vi "ZoneVacCtrldPickDrop_2StepVac.vi"(4 "Position":enum16{"1", "2"}(ring), 5 "VacuumState2":u8, 6 "Zone":enum16{"ZoneA", "ZoneB", "ZoneC", "ZoneD"}(ring), 7 "VacuumState1":u8, 8 "error in (no error)":errorcluster, 9 "controller in":refnum<k24>, 10 "Zspeed":dbl=50.0 format="%#_13g", 11 "Z":dbl=65.0) -> (0 "error out":errorcluster, 3 "controller out":refnum<k24>)   [LabVIEW 2019]
uses:
  C:/Users/TTUHEP/Documents/LabVIEW/Other Models/2010/Bin/Aerotech.A3200.dll
  Other Models/2010/Bin/Aerotech.A3200.dll
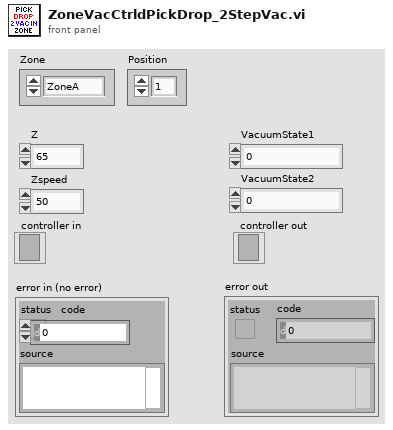
[diagram p1: front panel]
types:
  T1 = enum16{"BinarySwitch", "DecimalSwitch", "Conversion"}
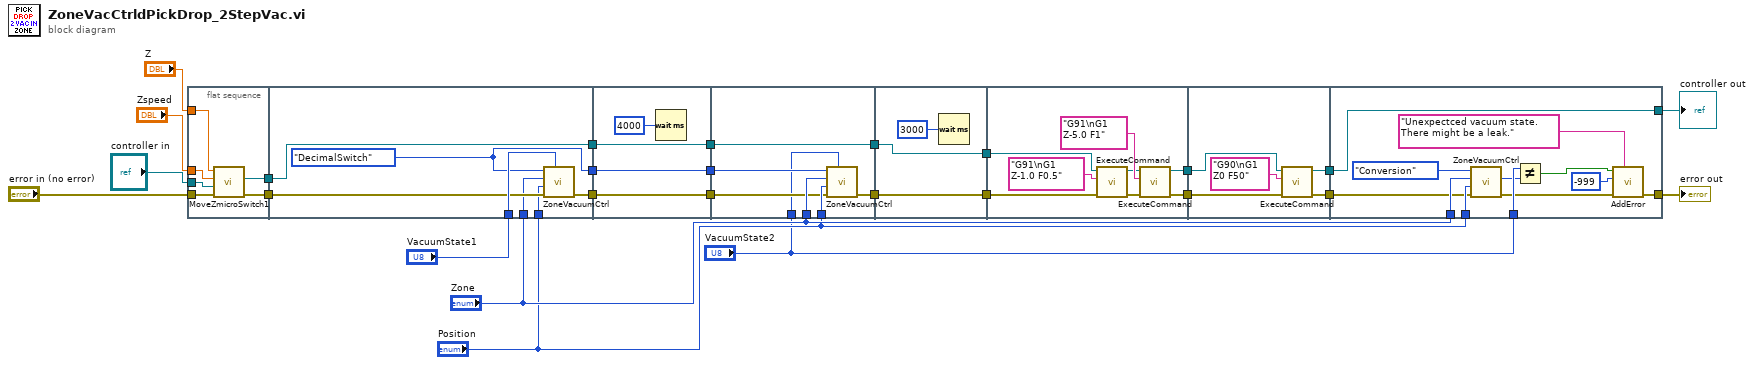
[diagram p0: block diagram]
diagram:
  n1 = flat-sequence {
    tunnel: [w29] -> w13
    tunnel: [w30] -> w12
    tunnel: "controller in" -> [w32]
    tunnel: "error in (no error)" -> [w31]
    tunnel: "Z" -> [w28]
    tunnel: "Zspeed" -> [w27]
    tunnel: w13 -> [w37]
    tunnel: [w34] -> w22
    tunnel: [w39] -> w21
    tunnel: w12 -> [w39]
    tunnel: "VacuumState1" -> [w38]
    tunnel: "Position" -> [w36]
    tunnel: "Zone" -> [w35]
    tunnel: [w33] -> w9
    tunnel: w22 -> [w43]
    tunnel: [w43] -> w11
    tunnel: w21 -> [w42]
    tunnel: [w42] -> w10
    tunnel: w9 -> [w40]
    tunnel: [w40] -> w8
    tunnel: w11 -> [w46]
    tunnel: [w45] -> w5
    tunnel: w10 -> [w50]
    tunnel: [w50] -> w3
    tunnel: w8 -> [w49]
    tunnel: "Zone" -> [w48]
    tunnel: "Position" -> [w47]
    tunnel: "VacuumState2" -> [w44]
    tunnel: w5 -> [w53]
    tunnel: [w53] -> w4
    tunnel: w3 -> [w52]
    tunnel: [w52] -> w2
    tunnel: w4 -> [w59]
    tunnel: [w54] -> w17
    tunnel: w2 -> [w60]
    tunnel: [w55] -> w16
    tunnel: w17 -> [w66]
    tunnel: w16 -> [w64]
    tunnel: [w63] -> w20
    tunnel: [w62] -> w14
    tunnel: w20 -> [w75]
    tunnel: [w76] -> w19
    tunnel: [w75] -> w18
    tunnel: "VacuumState2" -> [w74]
    tunnel: w14 -> [w70]
    tunnel: "Position" -> [w73]
    tunnel: "Zone" -> [w72]
    frame #0 {
      n2 = call "MoveZmicroSwitch1.vi"("Z"=w28, "Zspeed"=w27, "controller in"=w32, "error in (no error)"=w31) -> ("controller out"=w30:refnum<k24>, "error out"=w29:errorcluster)  [unwired: 3 in, 2 out]
    }
    frame #1 {
      w33 = T1."DecimalSwitch" ("ControlType")
      n3 = call "ZoneVacuumCtrl.vi"("DecimalIn"=w38, "Error In"=w37, "Position"=w36, "Zone"=w35, "ControlType"=w33) -> ("Error Out"=w34:errorcluster)  [unwired: 2 in, 4 out]
    }
    frame #2 {
      n4 = Wait (ms)(milliseconds to wait=u32 4000) -> ()  [unwired: 1 out]
    }
    frame #3 {
      n5 = call "ZoneVacuumCtrl.vi"("DecimalIn"=w44, "Error In"=w46, "Position"=w47, "Zone"=w48, "ControlType"=w49) -> ("Error Out"=w45:errorcluster)  [unwired: 2 in, 4 out]
    }
    frame #4 {
      n6 = Wait (ms)(milliseconds to wait=u32 3000) -> ()  [unwired: 1 out]
    }
    frame #5 {
      n7 = call "ExecuteCommand.vi"("error in (no error)"=w59, "Command Code"="G91\nG1 Z-1.0 F0.5", "controller in"=w60) -> ("error out"=w56:errorcluster, "controller out"=w57:refnum<k24>)  [unwired: 6 in, 1 out]
      n8 = call "ExecuteCommand.vi"("error in (no error)"=w56, "Command Code"="G91\nG1 Z-5.0 F1", "controller in"=w57) -> ("error out"=w54:errorcluster, "controller out"=w55:refnum<k24>)  [unwired: 6 in, 1 out]
    }
    frame #6 {
      n9 = call "ExecuteCommand.vi"("error in (no error)"=w66, "Command Code"="G90\nG1 Z0 F50", "controller in"=w64) -> ("error out"=w62:errorcluster, "controller out"=w63:refnum<k24>)  [unwired: 6 in, 1 out]
    }
    frame #7 {
      n10 = call "ZoneVacuumCtrl.vi"("Error In"=w70, "Position"=w73, "Zone"=w72, "ControlType"=T1."Conversion") -> ("Error Out"=w71:errorcluster, "DecimalOut"=w68:u32)  [unwired: 3 in, 3 out]
      n11 = Not Equal?(x=w74, y=w68) -> (x != y?=w67:bool)
      n12 = call "AddError.vi"("ErrorMessage"="Unexpectced vacuum state. There might be a leak.", "error in"=w71, "code"=-999, "Error?"=w67) -> ("Error out"=w76:errorcluster)  [unwired: 7 in]
    }
  }
  "controller out" <- w18
  "error out" <- w19
